vi "Add Sections and Leaves.vi"(6 "VS Refs":T1[](array[typedef]) format="%.0x", 8 "error in (no error)":errorcluster, 9 "LUT":variant, 10 "Items":string[](array[string]), 11 "TreeControl in":refnum<vi>) -> (0 "error out":errorcluster)   [LabVIEW 2013, in "OPC UA Client System Explorer.lvlib"]
uses:
  OPC UA Client System Explorer.lvlib
  <vilib>/NI Veristand/Custom Device API/Custom Device Item Ref.ctl
  <vilib>/NI Veristand/Custom Device API/Custom Device Channel.ctl
  <vilib>/NI Veristand/Custom Device API/Custom Device Channel Type.ctl
  Shared/Constants.vi
  <vilib>/NI Veristand/Custom Device API/Set Item Property (U32).vi
  <vilib>/NI Veristand/Custom Device API/Set Item Property (String).vi
  <vilib>/NI Veristand/Custom Device API/Custom Device API.lvlib
  Shared/OPC UA Client Shared.lvlib
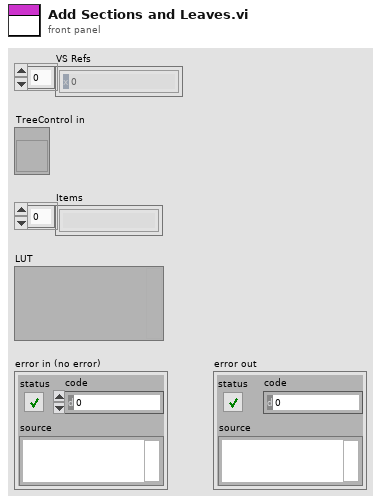
[diagram p1: front panel]
types:
  T1 = typedef "Custom Device API.lvlib/Custom Device Item Ref.ctl" = u64
  T2 = cluster{"name":string, "node type":enum32{"Other", "Folder", "Item/Property"}, "DataType":u32, "access":enum16{"Null", "Read", "Write", "Read&Write"}, "description":string}
  T3 = typedef "Custom Device API.lvlib/Custom Device Channel.ctl" = cluster{"Type":T4, "Units":string, "Default Value":dbl, "Faultable":bool, "Scalable":bool}
  T4 = typedef "Custom Device API.lvlib/Custom Device Channel Type.ctl" = enum16{"Input", "Output"}
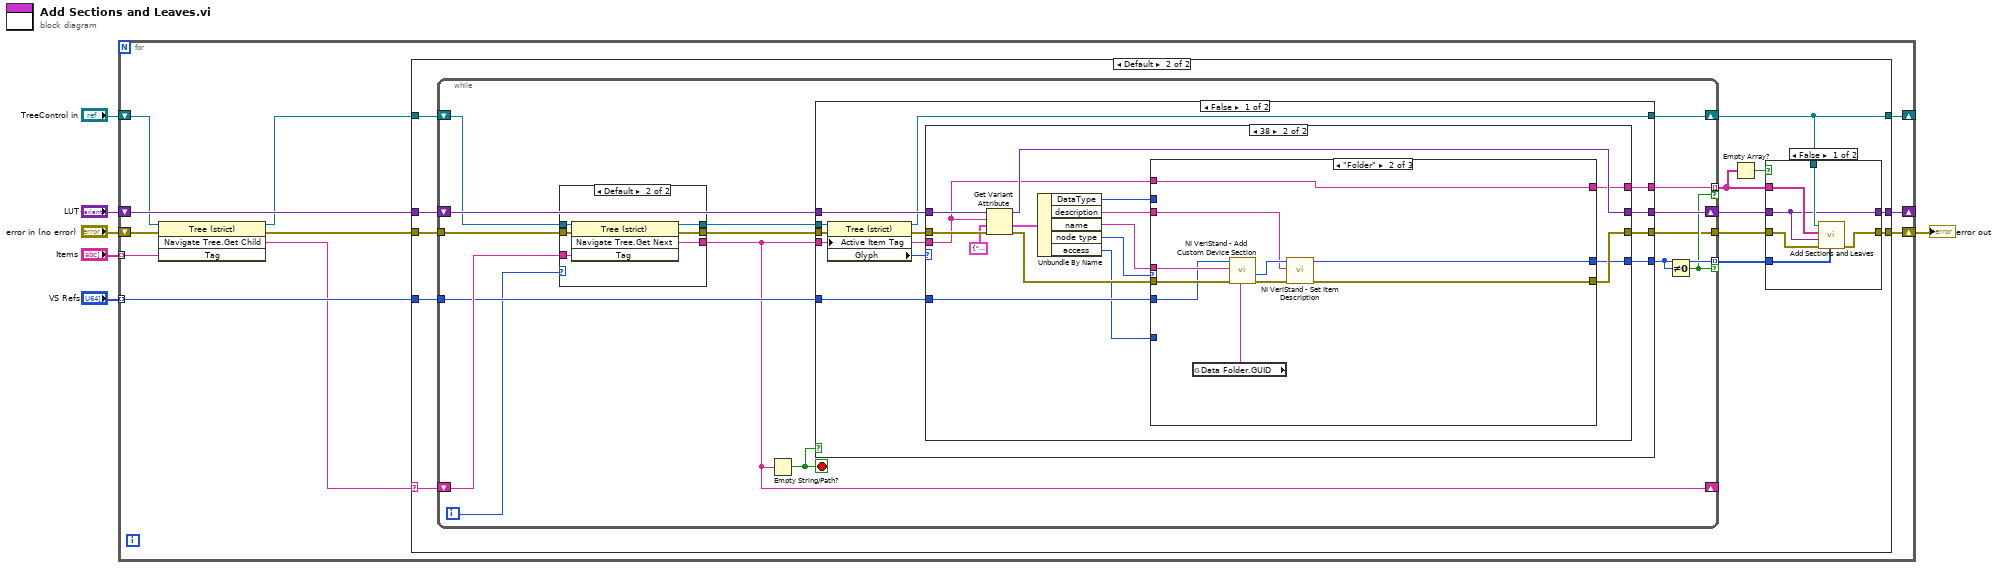
[diagram p0: block diagram]
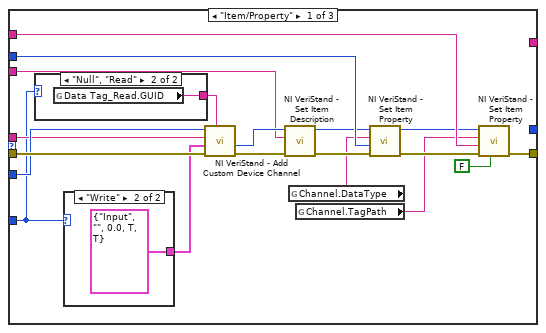
[diagram p6: hidden frame]
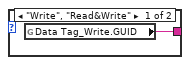
[diagram p7: hidden frame]
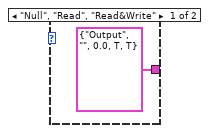
[diagram p8: hidden frame]
diagram:
  n1 = for {
    tunnel: "Items" -> [w8] mode=indexing
    tunnel: "VS Refs" -> [w17] mode=indexing
    shift-right: [w14] -> w1
    shift-left: "error in (no error)" -> [w12]
    shift-right: [w13] -> _
    shift-left: "LUT" -> [w16]
    shift-right: [w15] -> _
    shift-left: "TreeControl in" -> [w10]
    n2 = invoke class="Tree (strict)" method="Navigate Tree.Get Child"(reference=w10, error in=w12, "Tag"=w8) -> (reference out=w9:refnum<vi>, error out=w11:errorcluster, "Navigate Tree:Get Child"=w7:string)  [unwired: 1 in, 1 out]
    n3 = case shown="Default" w7 {
      selector: w7 -> [_ w21]
      tunnel: w17 -> [_ w33]
      tunnel: w16 -> [w19 w32]
      tunnel: [w20 w31] -> w15
      tunnel: [w18 w28] -> w14
      tunnel: [w19 w24] -> w13
      tunnel: w11 -> [w18 w23]
      tunnel: w9 -> [w20 w22]
      frame "" {
      }
      frame Default {
        n4 = while {
          tunnel: w23 -> [w56]
          shift-right: [w53] -> w30
          shift-left: w32 -> [w57]
          tunnel: [w51] -> w29 mode=indexing if=w49
          tunnel: [w50] -> w26 mode=indexing if=w49
          tunnel: w33 -> [w47]
          tunnel: [w46] -> w27
          shift-right: [w45] -> w31
          shift-left: w22 -> [w44]
          shift-right: [w43] -> _
          shift-left: w21 -> [w48]
          i -> [w42]
          stop <- w52 stop-if-true
          n5 = case shown="Default" w42 {
            tunnel: w56 -> [w59 w66]
            tunnel: [w58 w65] -> w55
            tunnel: [w59 w64] -> w54
            tunnel: w48 -> [w60 w63]
            tunnel: w44 -> [w58 w62]
            tunnel: [w60 w61] -> w43
            frame 0 {
            }
            frame Default {
              n6 = invoke class="Tree (strict)" method="Navigate Tree.Get Next"(reference=w62, error in=w66, "Tag"=w63) -> (reference out=w65:refnum<vi>, error out=w64:errorcluster, "Navigate Tree:Get Next Item"=w61:string)  [unwired: 1 in, 1 out]
            }
          }
          n7 = Empty String/Path?(string/path=w43) -> (empty?=w52:bool)
          n8 = case shown="False" w52 {
            tunnel: w57 -> [w78 w132]
            tunnel: w55 -> [w77 w131]
            tunnel: w54 -> [w76 w133]
            tunnel: w43 -> [w73 _]
            tunnel: [w72 w132] -> w53
            tunnel: [w71 w133] -> w46
            tunnel: [w70 _] -> w51
            tunnel: [w69 _] -> w50
            tunnel: w47 -> [w68 _]
            tunnel: [w67 w131] -> w45
            frame False {
              n9 = property class="Tree (strict)"(reference=w77, error in=w76, "Active Item Tag"=w73) -> (reference out=w67:refnum<vi>, error out=w75:errorcluster, "Glyph"=w74:i32)
              n10 = case shown="38" w74 {
                tunnel: w78 -> [w79 w96]
                tunnel: [w79 w95] -> w72
                tunnel: w75 -> [w80 w94]
                tunnel: w73 -> [_ w89]
                tunnel: [w80 w91] -> w71
                tunnel: [_ w90] -> w70
                tunnel: [_ w88] -> w69
                tunnel: w68 -> [_ w87]
                frame Default {
                }
                frame 38 {
                  n11 = Get Variant Attribute(Variant=w96, name=w89, default value (empty Variant)=T2 {"name"="", "node type"=enum."Other", "DataType"=1, "access"=enum."Null", "description"=""} ("node attribute"), error in=w94) -> (duplicate Variant=w95:variant, value=w92:T2, error out=w93:errorcluster)  [unwired: 1 out]
                  n12 = Unbundle By Name(w92) -> ("DataType"=w82:u32, "description"=w83:string, "name"=w85:string, "node type"=w84:enum32{"Other", "Folder", "Item/Property"}, "access"=w81:enum16{"Null", "Read", "Write", "Read&Write"})
                  n13 = case shown="\"Folder\"" w84 {
                    tunnel: w85 -> [w113 w129 _]
                    tunnel: w93 -> [w115 w128 w130]
                    tunnel: [_ w122 _] -> w90
                    tunnel: [w109 w124 w130] -> w91
                    tunnel: [_ w127 _] -> w88
                    tunnel: w89 -> [w108 w127 _]
                    tunnel: w87 -> [w114 w126 _]
                    tunnel: w83 -> [w110 w121 _]
                    tunnel: w82 -> [w107 _ _]
                    tunnel: w81 -> [w98 _ _]
                    frame "Item/Property" {
                      n14 = case shown="\"Null\", \"Read\"" w98 {
                        tunnel: [w116 w117] -> w97
                        frame "Write", "Read&Write" {
                          n15 = global read "Constants.vi" "Data Tag_Write.GUID"() -> (w116:string)
                        }
                        frame "Null", "Read" {
                          n16 = global read "Constants.vi" "Data Tag_Read.GUID"() -> (w117:string)
                        }
                      }
                      n17 = case shown="\"Write\"" w98 {
                        tunnel: [T3 {"Type"=enum."Output", "Units"="", "Default Value"=0.0, "Faultable"=TRUE, "Scalable"=TRUE} ("Channel") T3 {"Type"=enum."Input", "Units"="", "Default Value"=0.0, "Faultable"=TRUE, "Scalable"=TRUE} ("Channel")] -> w102
                        frame "Null", "Read", "Read&Write" {
                        }
                        frame "Write" {
                        }
                      }
                      n18 = call <vilib>:"NI VeriStand - Add Custom Device Channel.vi"("GUID (Default Channel)"=w97, "error in (no error)"=w115, "Channel"=w102, "Channel Name"=w113, "Parent Ref in"=w114) -> ("error out"=w112:errorcluster, "Channel Ref"=w111:T1)  [unwired: 3 in, 2 out]
                      n19 = call <vilib>:"NI VeriStand - Set Item Description.vi"("error in (no error)"=w112, "Description"=w110, "Item Ref in"=w111) -> ("error out"=w105:errorcluster, "Item Ref out"=w103:T1)  [unwired: 6 in, 1 out]
                      n20 = global read "Constants.vi" "Channel.DataType"() -> (w101:string)
                      n21 = global read "Constants.vi" "Channel.TagPath"() -> (w100:string)
                      n22 = call-poly <vilib>:"NI VeriStand - Set Item Property.vi"("error in (no error)"=w105, "Value"=w107, "Property Name"=w101, "Item Ref in"=w103) -> ("error out"=w104:errorcluster, "Item Ref out"=w106:T1)  [unwired: 5 in, 1 out]
                      n23 = call-poly <vilib>:"NI VeriStand - Set Item Property.vi"("Binary String (T)"=FALSE, "error in (no error)"=w104, "Value"=w108, "Property Name"=w100, "Item Ref in"=w106) -> ("error out"=w109:errorcluster)  [unwired: 4 in, 2 out]
                    }
                    frame "Folder" {
                      n24 = global read "Constants.vi" "Data Folder.GUID"() -> (w120:string)
                      n25 = call <vilib>:"NI VeriStand - Add Custom Device Section.vi"("GUID (Default Section)"=w120, "error in (no error)"=w128, "Section Name"=w129, "Parent Ref in"=w126) -> ("error out"=w125:errorcluster, "Section Ptr"=w123:T1)  [unwired: 4 in, 2 out]
                      n26 = call <vilib>:"NI VeriStand - Set Item Description.vi"("error in (no error)"=w125, "Description"=w121, "Item Ref in"=w123) -> ("error out"=w124:errorcluster, "Item Ref out"=w122:T1)  [unwired: 6 in, 1 out]
                    }
                    frame "Other" {
                    }
                  }
                }
              }
            }
            frame True {
            }
          }
          n27 = Not Equal To 0?(x=w51) -> (x != 0?=w49:bool)
        }
        n28 = Empty Array?(array=w26) -> (empty?=w25:bool)
        n29 = case shown="False" w25 {
          tunnel: w31 -> [w39 _]
          tunnel: w26 -> [w38 _]
          tunnel: w30 -> [w34 w40]
          tunnel: w29 -> [w37 _]
          tunnel: [w36 w41] -> w28
          tunnel: w27 -> [w35 w41]
          tunnel: [w34 w40] -> w24
          frame False {
            n30 = call "Add Sections and Leaves.vi"("VS Refs"=w37, "error in (no error)"=w35, "LUT"=w34, "Items"=w38, "TreeControl in"=w39) -> ("error out"=w36:errorcluster)  [unwired: 6 in]
          }
          frame True {
          }
        }
      }
    }
  }
  "error out" <- w1
